vi "Get_local_ADAM_Chs.vi"(2 "Local ADAM?":bool, 3 "Show setup":bool, 4 "Desired Local ADAM Channels":string[](array[string])) -> (0 "Chosen Channels":string[](array[string]), 1 "Ch Indicies Chosen":i32[](array[numeric]))   [LabVIEW 2016]
uses:
  ADAM Client/Sub VIs/ADAM Controls/Channel_names.ctl
  Globals/Constants_global.vi
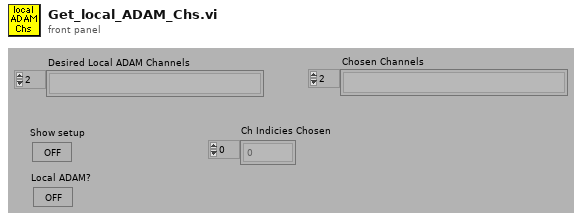
[diagram p1: front panel]
types:
  T1 = typedef "Channel_names.ctl" = enum16{"Active Only", "Active + Off", "All Channels"}
  T2 = enum16{"Zero or one", "One", "Zero or more", "One or more"}
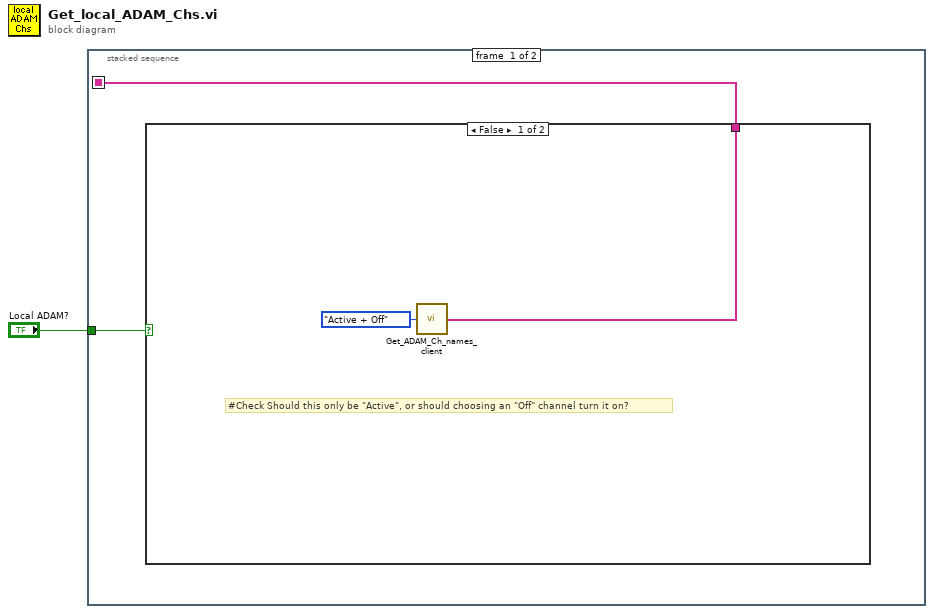
[diagram p0: block diagram]
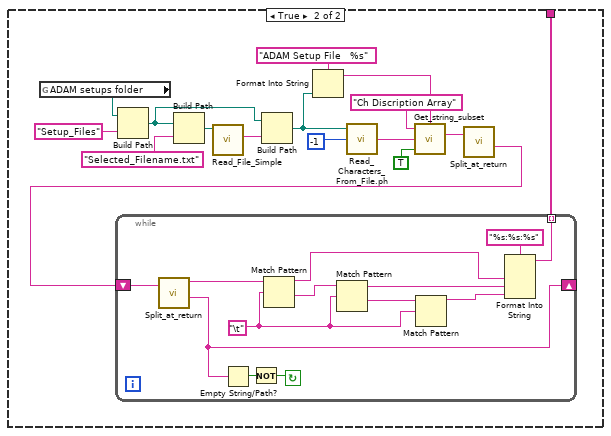
[diagram p2: hidden frame]
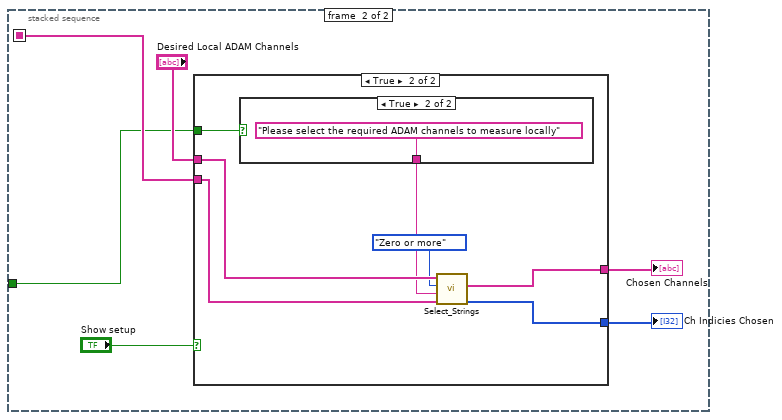
[diagram p3: hidden frame]
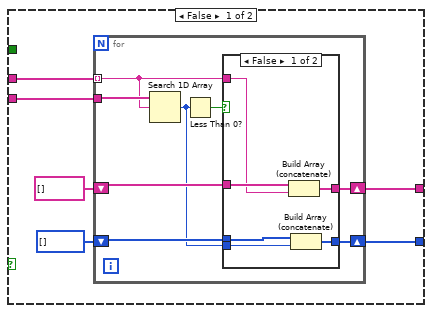
[diagram p4: hidden frame]
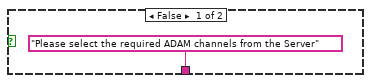
[diagram p6: hidden frame]
diagram:
  n1 = stacked-sequence {
    seq-local: [w3 _] -> [_ w40]
    tunnel: "Local ADAM?" -> [w2 w35]
    frame #0 {
      n2 = case shown="False" w2 {
        tunnel: [w4 w16] -> w3
        frame False {
          # "#Check Should this only be \"Active\", or should choosing an \"Off\" channel turn it on?"
          n3 = call "Get_ADAM_Ch_names_client.vi"("Channel names set"=Channel_names."Active + Off") -> ("Ch names"=w4:string[])
        }
        frame True {
          n4 = global read "Constants_global.vi" "ADAM setups folder"() -> (w13:path)
          n5 = Build Path(base path=w13, name or relative path="Setup_Files") -> (appended path=w10:path)
          n6 = Build Path(base path=w10, name or relative path="Selected_Filename.txt" ("Substring")) -> (appended path=w12:path)
          n7 = call "Read_File_Simple.vi"("Filename"=w12) -> ("string"=w11:string)  [unwired: 2 in, 7 out]
          n8 = Build Path(base path=w10, name or relative path=w11) -> (appended path=w7:path)
          n9 = Format Into String(format string="ADAM Setup File   %s", w7) -> (resulting string=w6:string)  [unwired: 2 in, 1 out]
          n10 = call "Read_Characters_From_File.ph.vi"("file path (dialog if empty)"=w7, "number of characters (all:-1)"=-1) -> ("character string"=w21:string)  [unwired: 7 out]
          n11 = call "Get_string_subset.vi"("String Name"=w6, "Show Dialog?"=TRUE, "String to split"=w21, "File Label"="Ch Discription Array") -> ("Output string"=w9:string)  [unwired: 1 out]
          n12 = call "Split_at_return.vi"("String"=w9) -> ("after substring"=w17:string)  [unwired: 1 in, 3 out]
          n13 = while {
            tunnel: [w22] -> w16 mode=indexing
            shift-left: w17 -> [w34]
            shift-right: [w33] -> _
            stop <- w31 continue-if-true
            w27 = "\t"
            n14 = call "Split_at_return.vi"("String"=w34) -> ("before substring"=w30:string, "after substring"=w33:string)  [unwired: 1 in, 2 out]
            n15 = Empty String/Path?(string/path=w33) -> (empty?=w32:bool)
            n16 = Not(x=w32) -> (.not. x?=w31:bool)
            n17 = Match Pattern(string=w30, regular expression=w27) -> (before substring=w23:string, after substring=w29:string)  [unwired: 3 out]
            n18 = Match Pattern(string=w29, regular expression=w27) -> (before substring=w26:string, after substring=w28:string)  [unwired: 3 out]
            n19 = Match Pattern(string=w28, regular expression=w27) -> (before substring=w25:string)  [unwired: 4 out]
            n20 = Format Into String(format string="%s:%s:%s" ("Format String"), w23, w26, w25) -> (resulting string=w22:string)  [unwired: 2 in, 1 out]
          }
        }
      }
    }
    frame #1 {
      n21 = case shown="True" "Show setup" {
        tunnel: w40 -> [w45 w69]
        tunnel: "Desired Local ADAM Channels" -> [w46 w68]
        tunnel: [w43 w65] -> w38
        tunnel: [w41 w66] -> w36
        tunnel: w35 -> [_ w63]
        frame False {
          n22 = for {
            tunnel: w45 -> [w54]
            tunnel: w46 -> [w50] mode=indexing
            shift-right: [w51] -> w43
            shift-left: string[] [] -> [w52]
            shift-right: [w48] -> w41
            shift-left: i32[] [] -> [w49]
            n23 = Search 1D Array(1D array=w54, element=w50) -> (index of element=w47:i32)  [unwired: 1 out]
            n24 = Less Than 0?(x=w47) -> (x < 0?=w53:bool)
            n25 = case shown="False" w53 {
              tunnel: w52 -> [w60 w62]
              tunnel: [w59 w62] -> w51
              tunnel: w50 -> [w58 _]
              tunnel: w49 -> [w57 w61]
              tunnel: [w56 w61] -> w48
              tunnel: w47 -> [w55 _]
              frame False {
                n26 = Build Array (concatenate)(w60, w58) -> (w59:string[])
                n27 = Build Array (concatenate)(w57, w55) -> (w56:i32[])
              }
              frame True {
              }
            }
          }
        }
        frame True {
          n28 = case shown="True" w63 {
            tunnel: ["Please select the required ADAM channels from the Server" ("Message") "Please select the required ADAM channels to measure locally" ("Message")] -> w67
            frame False {
            }
            frame True {
            }
          }
          n29 = call "Select_Strings.vi"("Available Ch names"=w69, "Message"=w67, "Selector mode"=T2."Zero or more", "Desired Ch names (in)"=w68) -> ("Ch Indicies Chosen"=w66:i32[], "Selected Channel Names"=w65:string[])  [unwired: 1 in, 2 out]
        }
      }
      "Chosen Channels" <- w38
      "Ch Indicies Chosen" <- w36
    }
  }
